vi "Select Color Brewer Palette v2.vi"(6 "User Choices":T2, 7 "Interpolate":bool, 8 "Error In":errorcluster, 9 "Color Ramp Refnum":refnum<vi>, 10 "Palette Colors":refnum<vi>, 11 "Palette List Refnum":refnum<vi>) -> (0 "Error Out":errorcluster, 1 "Palette Name":string, 2 "# Palettes":i32, 3 "Available Palettes":T1[](array[typedef]), 4 "Compatible Max # Colors":i32)   [LabVIEW 2021]
uses:
  Color Brewer Palette.ctl
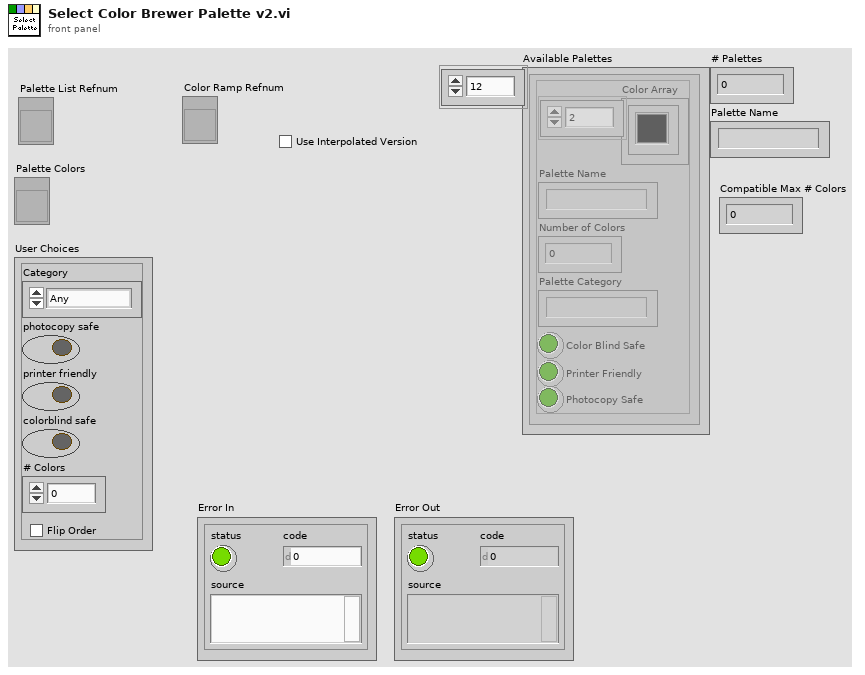
[diagram p1: front panel]
types:
  T1 = typedef "Color Brewer Palette.ctl" = cluster{"Color Array":u32[], "Palette Name":string, "Number of Colors":i32, "Palette Category":string, "Color Blind Safe":bool, "Printer Friendly":bool, "Photocopy Safe":bool}
  T2 = cluster{"Category":enum16{"Any", "Sequential", "Diverging", "Qualitative"}, "photocopy safe":bool, "printer friendly":bool, "colorblind safe":bool, "# Colors":i32, "Flip Order":bool}
  T3 = enum16{"Any", "Sequential", "Diverging", "Qualitative"}
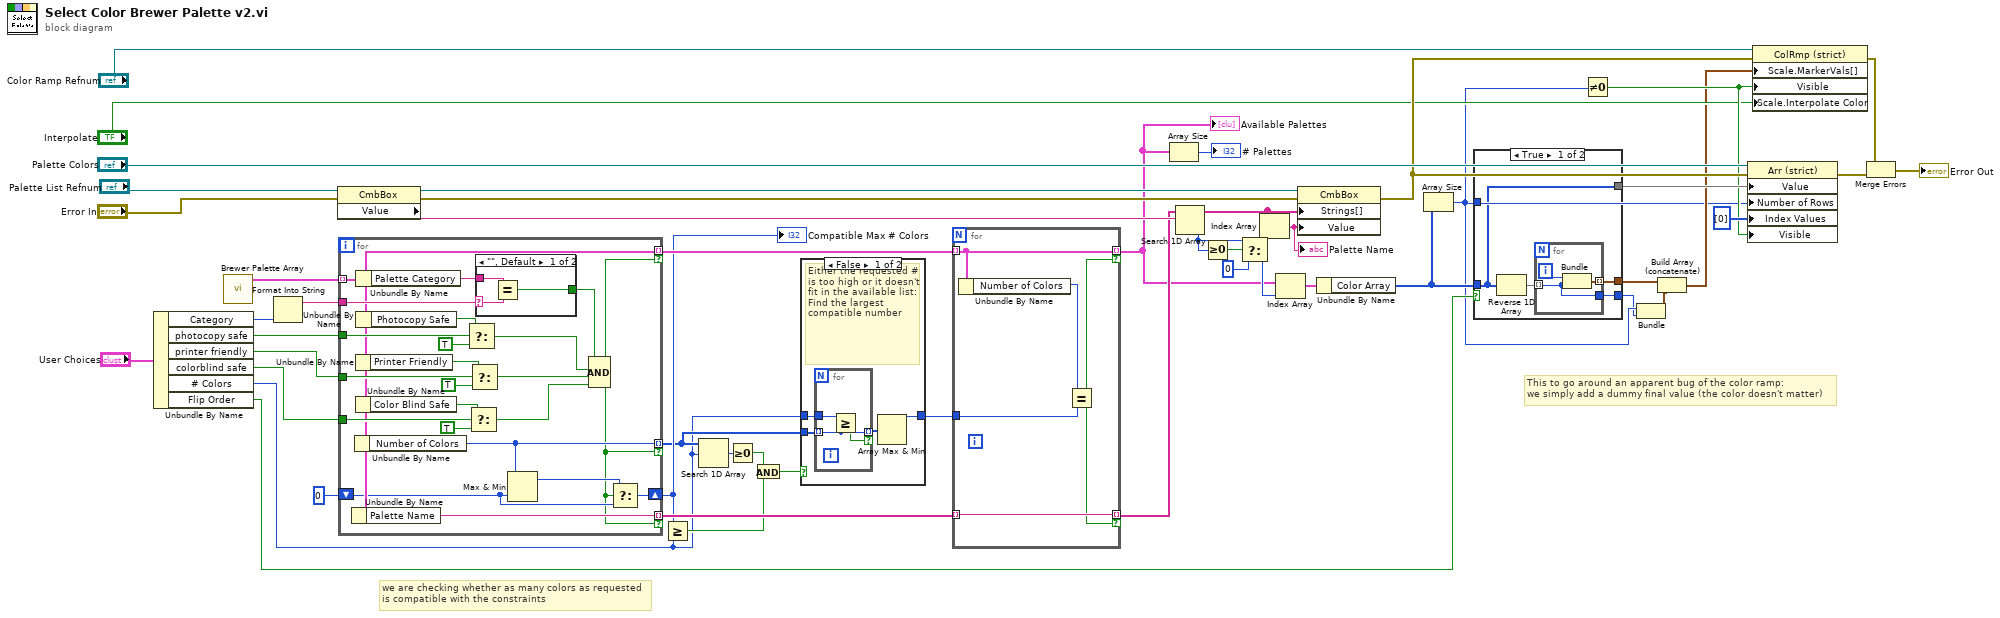
[diagram p0: block diagram]
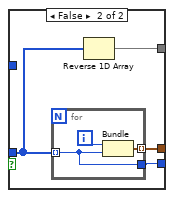
[diagram p3: hidden frame]
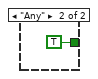
[diagram p4: hidden frame]
diagram:
  # "This to go around an apparent bug of the color ramp:\nwe simply add a dummy final value (the color doesn't matter)"
  # "we are checking whether as many colors as requested\nis compatible with the constraints"
  n1 = Unbundle By Name("User Choices") -> ("Category"=w47:T3, "photocopy safe"=w45:bool, "printer friendly"=w44:bool, "colorblind safe"=w43:bool, "# Colors"=w8:i32, "Flip Order"=w15:bool)
  n2 = call "Brewer Palette Array.vi"() -> ("Color Brewer Palette Array"=w48:T1[])  [unwired: 9 in]
  n3 = Format Into String(w47) -> (resulting string=w46:string)  [unwired: 3 in, 1 out]
  n4 = property class="CmbBox"(reference="Palette List Refnum", error in="Error In") -> (reference out=w36:refnum<vi>, error out=w34:errorcluster, "Value"=w33:string)
  n5 = for {
    tunnel: w48 -> [w56] mode=indexing
    tunnel: w46 -> [w70]
    tunnel: w45 -> [w69]
    tunnel: w44 -> [w64]
    tunnel: w43 -> [w61]
    tunnel: [w56] -> w18 mode=indexing if=w50
    tunnel: [w55] -> w17 mode=indexing if=w50
    shift-right: [w52] -> w14
    shift-left: 0 ("Number of Colors") -> [w53]
    tunnel: [w51] -> w9 mode=indexing if=w50
    n6 = Unbundle By Name(w56) -> ("Palette Name"=w55:string)
    n7 = Unbundle By Name(w56) -> ("Number of Colors"=w51:i32)
    n8 = Unbundle By Name(w56) -> ("Printer Friendly"=w65:bool)
    n9 = Unbundle By Name(w56) -> ("Color Blind Safe"=w63:bool)
    n10 = Unbundle By Name(w56) -> ("Palette Category"=w71:string)
    n11 = Unbundle By Name(w56) -> ("Photocopy Safe"=w68:bool)
    n12 = Select(t=w68, s=w69, f=TRUE) -> (s? t:f=w59:bool)
    n13 = Select(t=w63, s=w61, f=TRUE) -> (s? t:f=w57:bool)
    n14 = Select(t=w65, s=w64, f=TRUE) -> (s? t:f=w58:bool)
    n15 = case shown="\"\", Default" w70 {
      selector: w70 -> [w73 _]
      tunnel: w71 -> [w74 _]
      tunnel: [w72 TRUE] -> w60
      frame "", Default {
        n16 = Equal?(x=w74, y=w73) -> (x = y?=w72:bool)
      }
      frame "Any" {
      }
    }
    n17 = Max & Min(x=w51, y=w53) -> (max(x,y)=w54:i32)  [unwired: 1 out]
    n18 = Compound Arithmetic op=AND(w60, w59, w58, w57) -> (w50:bool)
    n19 = Select(t=w54, s=w50, f=w53) -> (s? t:f=w52:i32)
  }
  "Compatible Max # Colors" <- w14
  n20 = Greater Or Equal?(x=w14, y=w8) -> (x >= y?=w11:bool)
  n21 = Search 1D Array(1D array=w9, element=w8) -> (index of element=w13:i32)  [unwired: 1 in]
  n22 = Greater Or Equal To 0?(x=w13) -> (x >= 0?=w12:bool)
  n23 = And(x=w12, y=w11) -> (x .and. y?=w10:bool)
  n24 = case shown="False" w10 {
    tunnel: w9 -> [w79 _]
    tunnel: w8 -> [w78 w83]
    tunnel: [w76 w83] -> w7
    frame False {
      # "Either the requested # is too high or it doesn't fit in the available list: Find the largest compatible number"
      n25 = for {
        tunnel: w79 -> [w81] mode=indexing
        tunnel: w78 -> [w82]
        tunnel: [w81] -> w77 mode=indexing if=w80
        n26 = Greater Or Equal?(x=w82, y=w81) -> (x >= y?=w80:bool)
      }
      n27 = Array Max & Min(array=w77) -> (max value=w76:i32)  [unwired: 3 out]
    }
    frame True {
      # "there is a palette with the requested # colors"
    }
  }
  n28 = for {
    tunnel: w18 -> [w86] mode=indexing
    tunnel: w17 -> [w87] mode=indexing
    tunnel: [w87] -> w16 mode=indexing if=w85
    tunnel: [w86] -> w5 mode=indexing if=w85
    tunnel: w7 -> [w84]
    n29 = Unbundle By Name(w86) -> ("Number of Colors"=w88:i32)
    n30 = Equal?(x=w88, y=w84) -> (x = y?=w85:bool)
  }
  "Available Palettes" <- w5
  n31 = Array Size(array=w5) -> (size(s)=→"# Palettes":i32)
  n32 = Search 1D Array(1D array=w16, element=w33) -> (index of element=w31:i32)  [unwired: 1 in]
  n33 = Greater Or Equal To 0?(x=w31) -> (x >= 0?=w32:bool)
  n34 = Select(t=w31, s=w32, f=0) -> (s? t:f=w29:i32)
  n35 = Index Array(array=w16, index=w29) -> (element=w28:string)
  "Palette Name" <- w28
  n36 = Index Array(array=w5, index=w29) -> (element=w40:T1)
  n37 = property class="CmbBox"(reference=w36, error in=w34, "Strings[]"=w16, "Value"=w28) -> (error out=w26:errorcluster)  [unwired: 1 out]
  n38 = Unbundle By Name(w40) -> ("Color Array"=w25:u32[])
  n39 = Array Size(array=w25) -> (size(s)=w2:i32)
  n40 = case shown="True" w15 {
    tunnel: w2 -> [_ _]
    tunnel: w25 -> [w92 w99]
    tunnel: [w91 w98] -> w24
    tunnel: [w92 w97] -> w21
    tunnel: [w89 w96] -> w1
    frame True {
      n41 = Reverse 1D Array(array=w92) -> (reversed array=w90:u32[])
      n42 = for {
        tunnel: w90 -> [w93] mode=indexing
        tunnel: [w94] -> w91 mode=indexing
        tunnel: [w93] -> w89
        i -> [w95]
        n43 = Bundle(w95, "Color Box"=w93) -> (w94:cluster{i32, "Color Box":u32})  [unwired: 1 in]
      }
    }
    frame False {
      n44 = for {
        tunnel: w99 -> [w100] mode=indexing
        tunnel: [w101] -> w98 mode=indexing
        tunnel: [w100] -> w96
        i -> [w102]
        n45 = Bundle(w102, "Color Box"=w100) -> (w101:cluster{i32, "Color Box":u32})  [unwired: 1 in]
      }
      n46 = Reverse 1D Array(array=w99) -> (reversed array=w97:u32[])
    }
  }
  n47 = Not Equal To 0?(x=w2) -> (x != 0?=w20:bool)
  n48 = Bundle(w2, "Color Box"=w1) -> (w3:cluster{i32, "Color Box":u32})  [unwired: 1 in]
  n49 = Build Array (concatenate)(w24, w3) -> (w4:cluster{i32, "Color Box":u32}[])
  n50 = property class="Arr (strict)"(reference="Palette Colors", error in=w26, "Value"=w21, "Number of Rows"=w2, "Index Values"=u32[] [0], "Visible"=w20) -> (error out=w39:errorcluster)  [unwired: 1 out]
  n51 = property class="ColRmp (strict)"(reference="Color Ramp Refnum", error in=w26, "Scale.MarkerVals[]"=w4, "Visible"=w20, "Scale.Interpolate Color"="Interpolate") -> (error out=w22:errorcluster)  [unwired: 1 out]
  n52 = Merge Errors(w22, w39) -> (→"Error Out":errorcluster)
